vi "HRTF-Process Frame.vi"(0 "Cal.Data In":T1, 7 "AI Waveforms":dbl[][](array[numeric]), 9 "First":bool, 11 "error in (no error)":errorcluster) -> (4 "Cal.Data Out":T1, 13 "Status":string, 14 "Finished":bool, 15 "error out":errorcluster)   [LabVIEW 2015]
uses:
  Typedefs/HRTF-Runtime Data.ctl
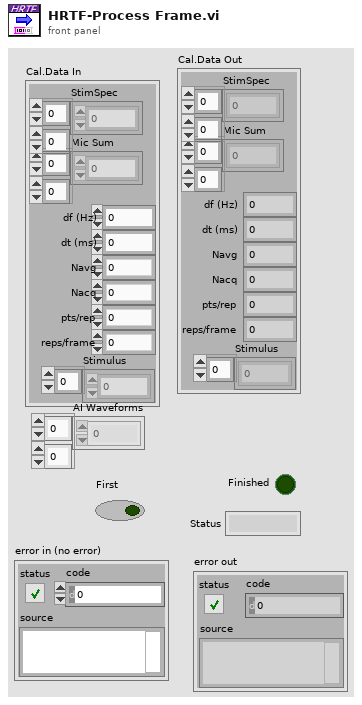
[diagram p1: front panel]
types:
  T1 = typedef "HRTF-Runtime Data.ctl" = cluster{"StimSpec":cdb[][], "Mic Sum":dbl[][], "df (Hz)":dbl, "dt (ms)":dbl, "Navg":i32, "Nacq":i32, "pts/rep":i32, "reps/frame":i32, "Stimulus":dbl[]}
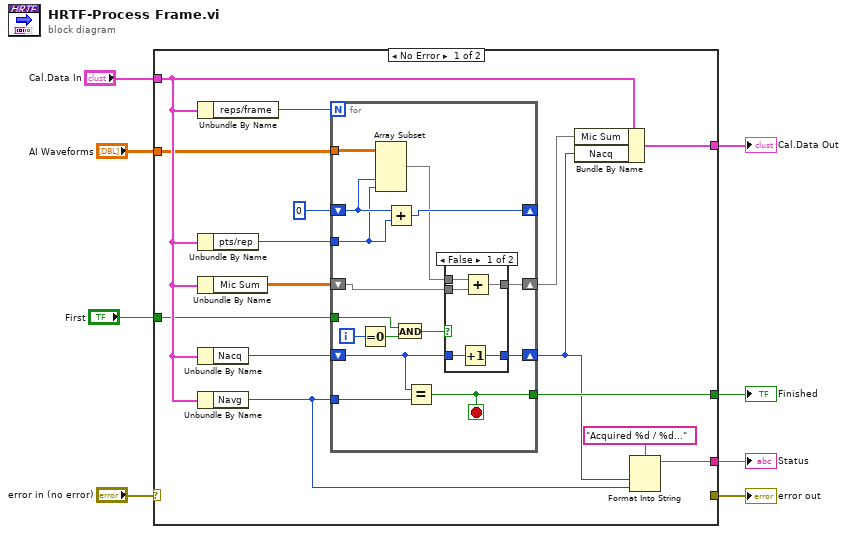
[diagram p0: block diagram]
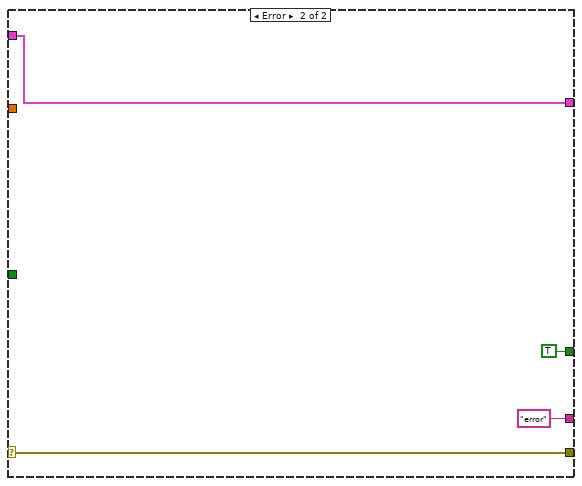
[diagram p3: hidden frame]
diagram:
  n1 = case shown="No Error" "error in (no error)" {
    selector: "error in (no error)" -> [_ w48]
    tunnel: "Cal.Data In" -> [w18 w49]
    tunnel: [w17 TRUE] -> w7
    tunnel: [w15 w49] -> w6
    tunnel: [_ w48] -> w4
    tunnel: [w13 "error"] -> w3
    tunnel: "AI Waveforms" -> [w10 _]
    tunnel: "First" -> [w9 _]
    frame No Error {
      n2 = Unbundle By Name(w18) -> ("reps/frame"=w22:i32)
      n3 = Unbundle By Name(w18) -> ("pts/rep"=w20:i32)
      n4 = Unbundle By Name(w18) -> ("Mic Sum"=w23:dbl[][])
      n5 = Unbundle By Name(w18) -> ("Nacq"=w19:i32)
      n6 = Unbundle By Name(w18) -> ("Navg"=w11:i32)
      n7 = for {
        N: w22 -> [_]
        shift-right: [w33] -> w16
        shift-left: w23 -> [w34]
        tunnel: w10 -> [w38]
        shift-right: [w35] -> _
        shift-left: 0 -> [w37]
        tunnel: w20 -> [w36]
        shift-right: [w25] -> w12
        shift-left: w19 -> [w24]
        tunnel: w11 -> [w31]
        tunnel: [w30] -> w17
        tunnel: w9 -> [w27]
        i -> [w29]
        stop <- w30 stop-if-true
        n8 = Equal To 0?(x=w29) -> (x = 0?=w28:bool)
        n9 = Array Subset(array=w38, index (col)=w37, length (col)=w36) -> (w32:dbl[][])  [unwired: 2 in]
        n10 = Add(x=w37, y=w36) -> (x+y=w35:i32)
        n11 = And(x=w27, y=w28) -> (x .and. y?=w26:bool)
        n12 = Equal?(x=w24, y=w31) -> (x = y?=w30:bool)
        n13 = case shown="False" w26 {
          tunnel: w34 -> [w43 w45]
          tunnel: [w42 w45] -> w33
          tunnel: w32 -> [w41 _]
          tunnel: w24 -> [w40 w44]
          tunnel: [w39 w44] -> w25
          frame False {
            n14 = Increment(x=w40) -> (x+1=w39:i32)
            n15 = Add(x=w41, y=w43) -> (x+y=w42:dbl[][])
          }
          frame True {
          }
        }
      }
      n16 = Bundle By Name(cluster=w18, "Mic Sum"=w16, "Nacq"=w12) -> (w15:T1)
      n17 = Format Into String(format string="Acquired %d / %d...", w12, w11) -> (resulting string=w13:string)  [unwired: 2 in, 1 out]
    }
    frame Error {
    }
  }
  "Cal.Data Out" <- w6
  "error out" <- w4
  "Status" <- w3
  "Finished" <- w7
